vi "Source-extraction-project.vi"() -> ()   [LabVIEW 2023]
panel:
  out "?":dbl(slide) scale=0.0..7000.0
  out "?":dbl(slide) scale=0.0..3000.0
  in  "STOP":bool
  out "Grid":bool
  out "renewable source":bool
  out "fuel cell":bool
  out "Battery":bool
  out "Wind Panel":bool
  out "Solar Panel":bool
  in  "Fuel cell":bool
  in  "Battery":bool
  in  "Wind turbine":bool
  in  "Solar PV":bool
  in  "Grid":bool
  out "Variable Load":dbl
  in  "Load Bank 3":bool
  in  "Load Bank 1":bool
  in  "Load Bank 2":bool
  out "Base Load":dbl
  in  "Motor 1":bool
  in  "Motor 2":bool
  # "Project Title :- Sources Extraction and Management Under Load Shedding Condition\n\nGuided by :-  Prof. S.S.Andhale \n\n   \n Name of Student :-\t\n                  1) Mantesh Aherwadi (B190312501)\n                  2)Ranjeet Hambire   (B190312548)\n                  3)Pranita Pachpande (B190312610)\n                  4)Yogesh Yangal  (B190312669)"
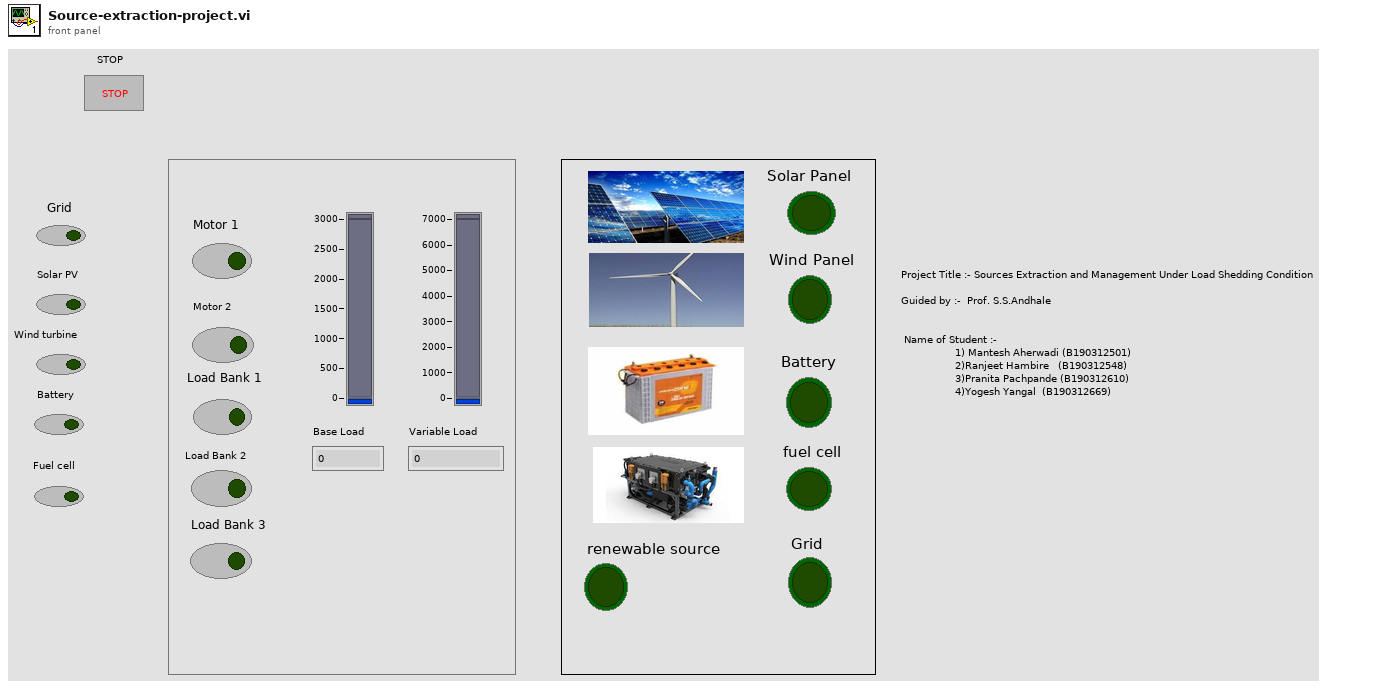
[diagram p1: front panel]
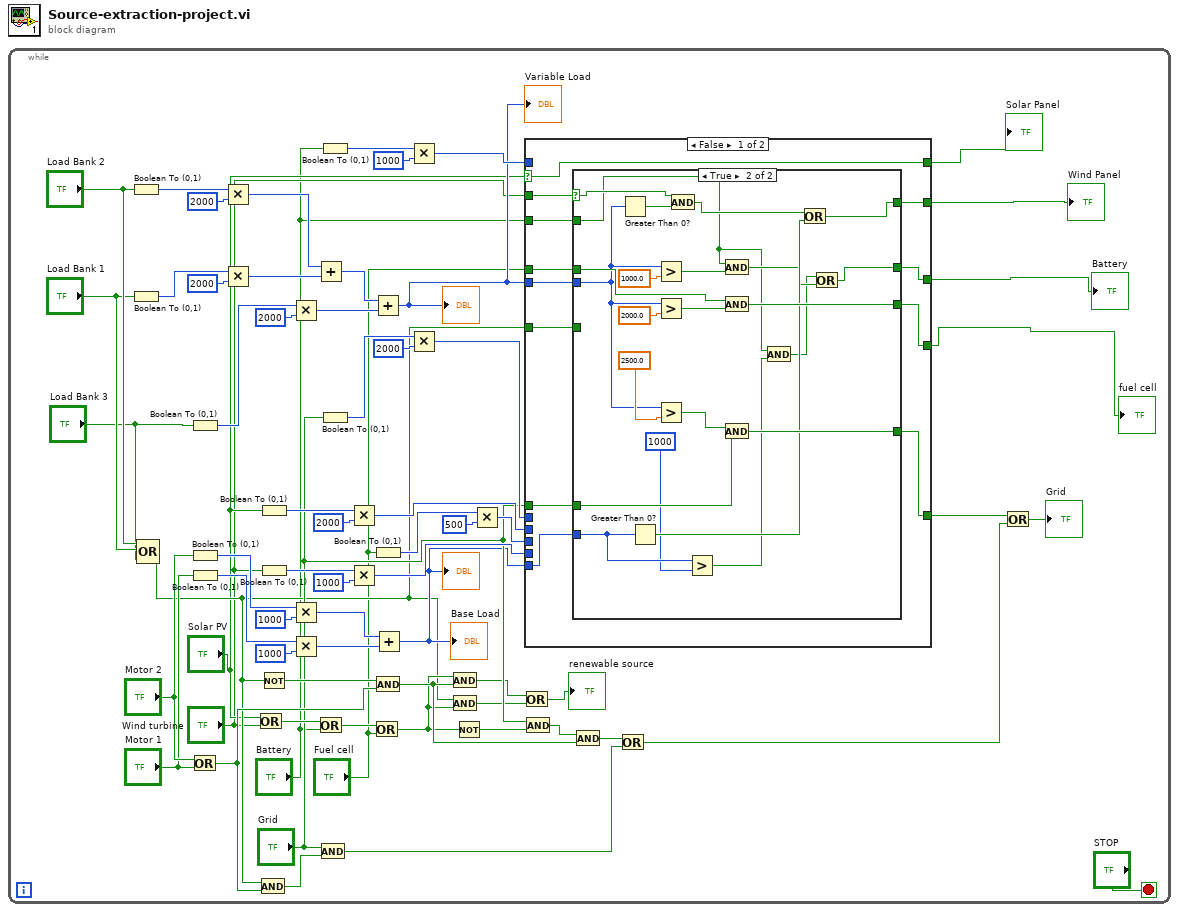
[diagram p0: block diagram]
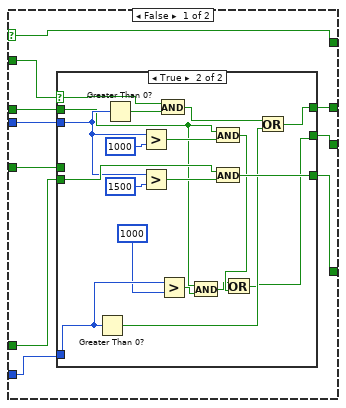
[diagram p2: hidden frame]
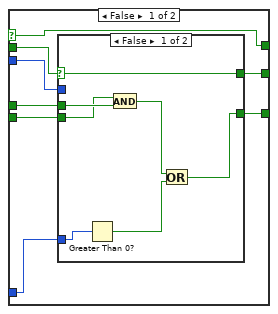
[diagram p3: hidden frame]
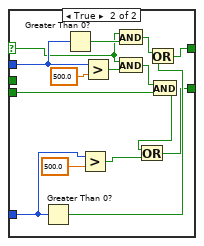
[diagram p4: hidden frame]
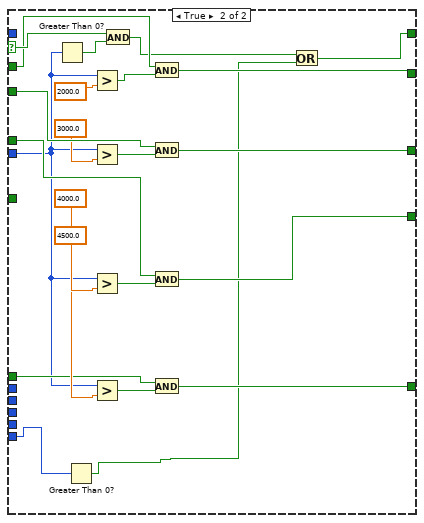
[diagram p5: hidden frame]
diagram:
  n1 = while {
    stop <- "STOP" stop-if-true
    n2 = Boolean To (0,1)(Boolean="Load Bank 2") -> (0, 1=w46:i16)
    n3 = Boolean To (0,1)(Boolean="Load Bank 1") -> (0, 1=w47:i16)
    n4 = Compound Arithmetic op=OR("Load Bank 2", "Load Bank 1", "Load Bank 3") -> (w10:bool)
    n5 = Boolean To (0,1)(Boolean="Load Bank 3") -> (0, 1=w43:i16)
    n6 = Boolean To (0,1)(Boolean="Motor 2") -> (0, 1=w50:i16)
    n7 = Boolean To (0,1)(Boolean="Motor 1") -> (0, 1=w51:i16)
    n8 = Or(x="Motor 2", y="Motor 1") -> (x .or. y?=w27:bool)
    n9 = Multiply(x=w46, y=i16 2000) -> (x*y=w45:i16)
    n10 = Multiply(x=w47, y=i16 2000) -> (x*y=w44:i16)
    n11 = Or(x="Solar PV", y="Wind turbine") -> (x .or. y?=w35:bool)
    n12 = And(x=w10, y=w27) -> (x .and. y?=w26:bool)
    n13 = Boolean To (0,1)(Boolean="Solar PV") -> (0, 1=w64:i16)
    n14 = Boolean To (0,1)(Boolean="Wind turbine") -> (0, 1=w62:i16)
    n15 = Not(x=w10) -> (.not. x?=w31:bool)
    n16 = Multiply(x=w43, y=i16 2000) -> (x*y=w42:i16)
    n17 = Multiply(x=w50, y=i16 1000) -> (x*y=w49:i16)
    n18 = Multiply(x=w51, y=i16 1000) -> (x*y=w48:i16)
    n19 = Add(x=w45, y=w44) -> (x+y=w41:i16)
    n20 = Or(x=w35, y="Battery") -> (x .or. y?=w34:bool)
    n21 = And(x="Grid", y=w26) -> (x .and. y?=w23:bool)
    n22 = Boolean To (0,1)(Boolean="Battery") -> (0, 1=w60:i16)
    n23 = Boolean To (0,1)(Boolean="Grid") -> (0, 1=w66:i16)
    n24 = Multiply(x=w64, y=i16 2000) -> (x*y=w37:i16)
    n25 = Multiply(x=w62, y=i16 1000) -> (x*y=w40:i16)
    n26 = Or(x=w34, y="Fuel cell") -> (x .or. y?=w22:bool)
    n27 = Add(x=w41, y=w42) -> (x+y=w14:i16)
    "Variable Load" <- w14
    "?" <- w14
    n28 = Boolean To (0,1)(Boolean="Fuel cell") -> (0, 1=w58:i16)
    n29 = And(x=w31, y=w27) -> (x .and. y?=w30:bool)
    n30 = Add(x=w49, y=w48) -> (x+y=w15:i16)
    "Base Load" <- w15
    "?" <- w15
    n31 = Multiply(x=w60, y=i16 1000) -> (x*y=w39:i16)
    n32 = Multiply(x=w66, y=i16 2000) -> (x*y=w36:i16)
    n33 = And(x=w22, y=w30) -> (x .and. y?=w20:bool)
    n34 = And(x=w10, y=w22) -> (x .and. y?=w21:bool)
    n35 = Not(x=w22) -> (.not. x?=w29:bool)
    n36 = Multiply(x=w58, y=i16 500) -> (x*y=w38:i16)
    n37 = Or(x=w20, y=w21) -> (x .or. y?=→"renewable source":bool)
    n38 = And(x="Grid", y=w29) -> (x .and. y?=w28:bool)
    n39 = case shown="False" "Solar PV" {
      selector: "Solar PV" -> [w68 w182]
      tunnel: "Wind turbine" -> [w78 w180]
      tunnel: "Fuel cell" -> [w76 w173]
      tunnel: w14 -> [w72 w165]
      tunnel: [w68 w162] -> w4
      tunnel: [w69 w179] -> w3
      tunnel: [w70 w176] -> w2
      tunnel: [w71 w172] -> w1
      tunnel: w15 -> [w67 w164]
      tunnel: w40 -> [_ _]
      tunnel: w39 -> [_ _]
      tunnel: w38 -> [_ _]
      tunnel: w37 -> [_ _]
      tunnel: "Grid" -> [w75 w169]
      tunnel: w36 -> [_ _]
      tunnel: "Battery" -> [w77 w177]
      tunnel: [w73 w168] -> w16
      tunnel: w10 -> [w74 _]
      frame False {
        n40 = case shown="True" w78 {
          selector: w78 -> [w80 w160]
          tunnel: w77 -> [w88 w139]
          tunnel: w76 -> [w87 w156]
          tunnel: w75 -> [w86 w153]
          tunnel: w74 -> [w85 _]
          tunnel: [w84 w152] -> w73
          tunnel: w72 -> [w83 w148]
          tunnel: [w82 w155] -> w71
          tunnel: [w81 w141] -> w70
          tunnel: [w80 w145] -> w69
          tunnel: w67 -> [w79 w144]
          frame False {
            n41 = case shown="True" w88 {
              selector: w88 -> [w90 w137]
              tunnel: w87 -> [w96 w119]
              tunnel: w86 -> [w95 w131]
              tunnel: w85 -> [w94 _]
              tunnel: [w93 w129] -> w84
              tunnel: w83 -> [w92 w130]
              tunnel: [w91 w122] -> w82
              tunnel: [w90 w126] -> w81
              tunnel: w79 -> [w89 w125]
              frame False {
                n42 = case shown="False" w96 {
                  selector: w96 -> [w101 w115]
                  tunnel: w95 -> [w102 w112]
                  tunnel: w94 -> [w103 _]
                  tunnel: [w97 w106] -> w93
                  tunnel: w92 -> [_ w116]
                  tunnel: [w101 w109] -> w91
                  tunnel: w89 -> [w100 w107]
                  frame False {
                    n43 = Greater Than 0?(x=w100) -> (x > 0?=w98:bool)
                    n44 = And(x=w102, y=w103) -> (x .and. y?=w99:bool)
                    n45 = Or(x=w99, y=w98) -> (x .or. y?=w97:bool)
                  }
                  frame True {
                    n46 = Greater Than 0?(x=w107) -> (x > 0?=w110:bool)
                    n47 = Greater Than 0?(x=w116) -> (x > 0?=w118:bool)
                    n48 = Greater?(x=w107, y=500.0) -> (0:w104:bool)
                    n49 = Greater?(x=w116, y=500.0) -> (0:w114:bool)
                    n50 = And(x=w115, y=w118) -> (x .and. y?=w111:bool)
                    n51 = And(x=w115, y=w114) -> (x .and. y?=w113:bool)
                    n52 = Or(x=w111, y=w110) -> (x .or. y?=w109:bool)
                    n53 = And(x=w113, y=w112) -> (x .and. y?=w105:bool)
                    n54 = Or(x=w105, y=w104) -> (x .or. y?=w106:bool)
                  }
                }
              }
              frame True {
                n55 = Greater Than 0?(x=w125) -> (x > 0?=w127:bool)
                n56 = Greater Than 0?(x=w130) -> (x > 0?=w136:bool)
                n57 = Greater?(x=w130, y=i16 1000) -> (0:w135:bool)
                n58 = Greater?(x=w130, y=i16 1500) -> (0:w133:bool)
                n59 = And(x=w137, y=w136) -> (x .and. y?=w128:bool)
                n60 = Greater?(x=w125, y=i16 1000) -> (0:w120:bool)
                n61 = And(x=w119, y=w120) -> (x .and. y?=w121:bool)
                n62 = And(x=w119, y=w135) -> (x .and. y?=w123:bool)
                n63 = And(x=w131, y=w133) -> (x .and. y?=w129:bool)
                n64 = Or(x=w121, y=w123) -> (x .or. y?=w122:bool)
                n65 = Or(x=w128, y=w127) -> (x .or. y?=w126:bool)
              }
            }
          }
          frame True {
            n66 = Greater Than 0?(x=w148) -> (x > 0?=w159:bool)
            n67 = Greater Than 0?(x=w144) -> (x > 0?=w146:bool)
            n68 = Greater?(x=w148, y=1000.0 ("x")) -> (0:w158:bool)
            n69 = Greater?(x=w148, y=2000.0 ("x")) -> (0:w157:bool)
            n70 = Greater?(x=w148, y=2500.0 ("x")) -> (0:w154:bool)
            n71 = And(x=w160, y=w159) -> (x .and. y?=w147:bool)
            n72 = Greater?(x=w144, y=i16 1000) -> (0:w140:bool)
            n73 = And(x=w139, y=w158) -> (x .and. y?=w142:bool)
            n74 = And(x=w156, y=w157) -> (x .and. y?=w155:bool)
            n75 = And(x=w154, y=w153) -> (x .and. y?=w152:bool)
            n76 = And(x=w139, y=w140) -> (x .and. y?=w138:bool)
            n77 = Or(x=w147, y=w146) -> (x .or. y?=w145:bool)
            n78 = Or(x=w138, y=w142) -> (x .or. y?=w141:bool)
          }
        }
      }
      frame True {
        n79 = Greater Than 0?(x=w165) -> (x > 0?=w183:bool)
        n80 = Greater Than 0?(x=w164) -> (x > 0?=w161:bool)
        n81 = Greater?(x=w165, y=2000.0 ("x")) -> (0:w181:bool)
        n82 = Greater?(x=w165, y=3000.0 ("x")) -> (0:w178:bool)
        n83 = Greater?(x=w165, y=4000.0) -> (0:w174:bool)
        n84 = Greater?(x=w165, y=4500.0) -> (0:w170:bool)
        n85 = And(x=w182, y=w183) -> (x .and. y?=w163:bool)
        n86 = And(x=w180, y=w181) -> (x .and. y?=w179:bool)
        n87 = And(x=w177, y=w178) -> (x .and. y?=w176:bool)
        n88 = And(x=w173, y=w174) -> (x .and. y?=w172:bool)
        n89 = And(x=w169, y=w170) -> (x .and. y?=w168:bool)
        n90 = Or(x=w163, y=w161) -> (x .or. y?=w162:bool)
      }
    }
    "Solar Panel" <- w4
    "Wind Panel" <- w3
    "Battery" <- w2
    "fuel cell" <- w1
    n91 = And(x=w28, y=w30) -> (x .and. y?=w24:bool)
    n92 = Or(x=w24, y=w23) -> (x .or. y?=w18:bool)
    n93 = Or(x=w16, y=w18) -> (x .or. y?=→"Grid":bool)
  }
